vi "Configure ARB Clipping.vi"(6 "Clipping Level2 (100 percent)":dbl=100.0, 7 "File Name (\"\")":string, 8 "error in (no error)":errorcluster, 9 "Clipping Level1 (100 percent)":dbl=100.0, 10 "Clipping Type (0: |I+jQ|)":u16(ring) items=["|I+jQ|", "|I|, |Q|"], 11 "VISA resource name":refnum<visa-resource-name>) -> (0 "error out":errorcluster, 3 "VISA resource name out":refnum<visa-resource-name>)   [LabVIEW 2012, in "Agilent PSG MXG Series.lvlib"]
doc: "Configures the clipping level of the waveform segment to a percentage of its highest peak.\n\n<B>Notes:</B>\n(1) This VI is valid only in E8267C, E8267D, N5162A, N5182A, N5172B, N5182B.\n\n(2) For E8267C, this VI is valid only when the instrument installs <B>Option 002</B> (Internal baseband generator) or <B>Option 602</B> (Digital bus baseband generator).\n\n(3) For E8267D, this VI is valid only when the instrument installs <B>Option 601</B> or <B>Option 602</B> (Internal baseband generator).\n\n(4) For N5162A and N5182A, this VI is valid only when the instrument installs <B>Option 651</B> or <B>Option 652</B> or <B>Option 654</B> (Internal baseband generator)."
uses:
  <instrlib>/Agilent PSG MXG Series/Agilent PSG MXG Series.lvlib
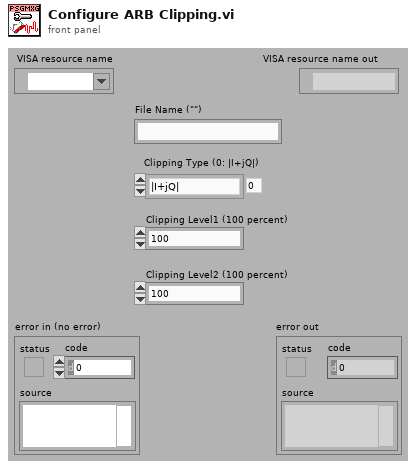
[diagram p1: front panel]
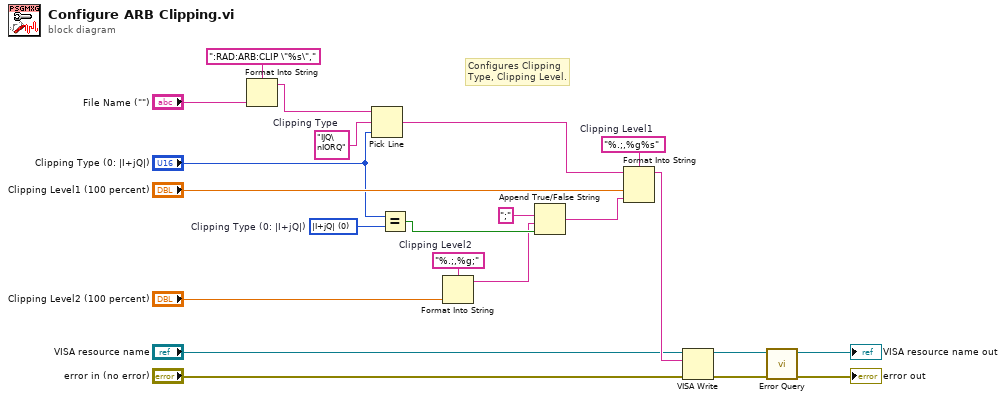
[diagram p0: block diagram]
diagram:
  w11 = u16 0 items=["|I+jQ|", "|I|, |Q|"]  # Clipping Type (0: |I+jQ|)
  w15 = "%.;,%g;"  # Clipping Level2
  w17 = "%.;,%g%s"  # Clipping Level1
  w19 = "IJQ\nIORQ"  # Clipping Type
  # "Configures Clipping\nType, Clipping Level."
  n1 = Format Into String(format string=":RAD:ARB:CLIP \"%s\",", "File Name (\"\")") -> (resulting string=w20:string)  [unwired: 2 in, 1 out]
  n2 = Pick Line(string ("")=w20, multi-line string=w19, line index="Clipping Type (0: |I+jQ|)") -> (output string=w18:string)
  n3 = Equal?(x="Clipping Type (0: |I+jQ|)", y=w11) -> (x = y?=w10:bool)
  n4 = Format Into String(format string=w15, "Clipping Level2 (100 percent)") -> (resulting string=w8:string)  [unwired: 2 in, 1 out]
  n5 = Append True/False String(1:w10, 2:w8, 3:";" ("false string")) -> (0:w13:string)  [unwired: 1 out]
  n6 = Format Into String(format string=w17, initial string=w18, "Clipping Level1 (100 percent)", w13) -> (resulting string=w7:string)  [unwired: 1 in, 1 out]
  n7 = VISA Write(VISA resource name="VISA resource name", write buffer=w7, error in (no error)="error in (no error)") -> (VISA resource name out=w6:refnum<visa-resource-name>, error out=w5:errorcluster)  [unwired: 1 out]
  n8 = call <instrlib>:"Error Query.vi"("error in (no error)"=w5, "VISA resource name"=w6) -> ("error out"=→"error out":errorcluster, "VISA resource name out"=→"VISA resource name out":refnum<visa-resource-name>)  [unwired: 8 out]
